vi "Shutdown.vi"(11 "Blueprint in":refnum<class "Blueprint.lvclass">) -> (2 "max geodes":u8, 3 "Blueprint out":refnum<class "Blueprint.lvclass">)   [LabVIEW 2023, in "d19.lvlib" / "Blueprint.lvclass"]
uses:
  Blueprint.lvclass
  Blueprint.lvclass/Blueprint.ctl
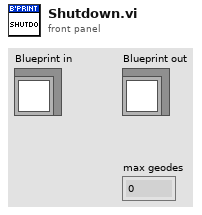
[diagram p1: front panel]
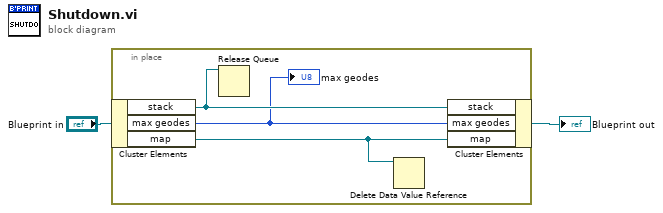
[diagram p0: block diagram]
diagram:
  n1 = in-place {
    n2 = in-place-cluster #1("Blueprint in") -> ("stack"=w5:refnum<queue>, "max geodes"=w4:u8, "map"=w3:refnum<data-value>)
    "max geodes" <- w4
    n3 = Release Queue(queue=w5) -> ()  [unwired: 2 in, 3 out]
    n4 = Delete Data Value Reference(data value reference=w3) -> ()  [unwired: 1 in, 2 out]
    n5 = in-place-cluster #1("stack"=w5, "max geodes"=w4, "map"=w3) -> (→"Blueprint out":refnum<class "Blueprint.lvclass">)
  }
